vi "Destroy_Timer_Ref.vi"   [LabVIEW 2018]
uses:
  Global/TimerReferences.vi
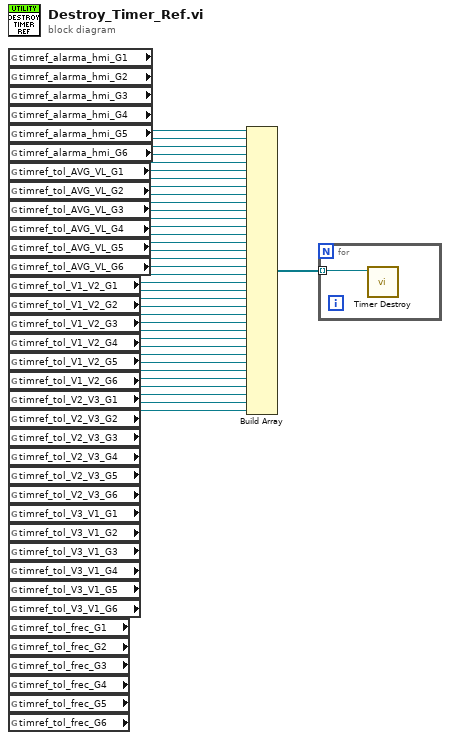
[diagram p0: block diagram]
diagram:
  n1 = global read "TimerReferences.vi" "timref_alarma_hmi_G1"() -> (w37:refnum<data-value>)
  n2 = global read "TimerReferences.vi" "timref_alarma_hmi_G2"() -> (w36:refnum<data-value>)
  n3 = global read "TimerReferences.vi" "timref_alarma_hmi_G3"() -> (w35:refnum<data-value>)
  n4 = global read "TimerReferences.vi" "timref_alarma_hmi_G4"() -> (w34:refnum<data-value>)
  n5 = global read "TimerReferences.vi" "timref_alarma_hmi_G5"() -> (w33:refnum<data-value>)
  n6 = global read "TimerReferences.vi" "timref_alarma_hmi_G6"() -> (w32:refnum<data-value>)
  n7 = global read "TimerReferences.vi" "timref_tol_AVG_VL_G1"() -> (w31:refnum<data-value>)
  n8 = global read "TimerReferences.vi" "timref_tol_AVG_VL_G2"() -> (w30:refnum<data-value>)
  n9 = global read "TimerReferences.vi" "timref_tol_AVG_VL_G3"() -> (w29:refnum<data-value>)
  n10 = global read "TimerReferences.vi" "timref_tol_AVG_VL_G4"() -> (w28:refnum<data-value>)
  n11 = global read "TimerReferences.vi" "timref_tol_AVG_VL_G5"() -> (w27:refnum<data-value>)
  n12 = global read "TimerReferences.vi" "timref_tol_AVG_VL_G6"() -> (w26:refnum<data-value>)
  n13 = global read "TimerReferences.vi" "timref_tol_V1_V2_G1"() -> (w25:refnum<data-value>)
  n14 = global read "TimerReferences.vi" "timref_tol_V1_V2_G2"() -> (w24:refnum<data-value>)
  n15 = global read "TimerReferences.vi" "timref_tol_V1_V2_G3"() -> (w23:refnum<data-value>)
  n16 = global read "TimerReferences.vi" "timref_tol_V1_V2_G4"() -> (w22:refnum<data-value>)
  n17 = global read "TimerReferences.vi" "timref_tol_V1_V2_G5"() -> (w21:refnum<data-value>)
  n18 = global read "TimerReferences.vi" "timref_tol_V1_V2_G6"() -> (w20:refnum<data-value>)
  n19 = global read "TimerReferences.vi" "timref_tol_V2_V3_G1"() -> (w19:refnum<data-value>)
  n20 = global read "TimerReferences.vi" "timref_tol_V2_V3_G2"() -> (w18:refnum<data-value>)
  n21 = global read "TimerReferences.vi" "timref_tol_V2_V3_G3"() -> (w17:refnum<data-value>)
  n22 = global read "TimerReferences.vi" "timref_tol_V2_V3_G4"() -> (w16:refnum<data-value>)
  n23 = global read "TimerReferences.vi" "timref_tol_V2_V3_G5"() -> (w15:refnum<data-value>)
  n24 = global read "TimerReferences.vi" "timref_tol_V2_V3_G6"() -> (w14:refnum<data-value>)
  n25 = global read "TimerReferences.vi" "timref_tol_V3_V1_G1"() -> (w13:refnum<data-value>)
  n26 = global read "TimerReferences.vi" "timref_tol_V3_V1_G2"() -> (w12:refnum<data-value>)
  n27 = global read "TimerReferences.vi" "timref_tol_V3_V1_G3"() -> (w11:refnum<data-value>)
  n28 = global read "TimerReferences.vi" "timref_tol_V3_V1_G4"() -> (w10:refnum<data-value>)
  n29 = global read "TimerReferences.vi" "timref_tol_V3_V1_G5"() -> (w9:refnum<data-value>)
  n30 = global read "TimerReferences.vi" "timref_tol_V3_V1_G6"() -> (w8:refnum<data-value>)
  n31 = global read "TimerReferences.vi" "timref_tol_frec_G1"() -> (w7:refnum<data-value>)
  n32 = global read "TimerReferences.vi" "timref_tol_frec_G2"() -> (w6:refnum<data-value>)
  n33 = global read "TimerReferences.vi" "timref_tol_frec_G3"() -> (w5:refnum<data-value>)
  n34 = global read "TimerReferences.vi" "timref_tol_frec_G4"() -> (w4:refnum<data-value>)
  n35 = global read "TimerReferences.vi" "timref_tol_frec_G5"() -> (w3:refnum<data-value>)
  n36 = global read "TimerReferences.vi" "timref_tol_frec_G6"() -> (w2:refnum<data-value>)
  n37 = Build Array(w37, w36, w35, w34, w33, w32, w31, w30, w29, w28, w27, w26, w25, w24, w23, w22, w21, w20, w19, w18, w17, w16, w15, w14, w13, w12, w11, w10, w9, w8, w7, w6, w5, w4, w3, w2) -> (w1:refnum<data-value>[])
  n38 = for {
    tunnel: w1 -> [w38] mode=indexing
    n39 = call "Timer Destroy.vi"("Timer reference"=w38) -> ()  [unwired: 10 in, 1 out]
  }
